vi "Read chat_model.vi"(8 "error in (no error)":errorcluster, 11 "agent_simple_qa in":refnum<class "agent_simple_qa.lvclass">) -> (0 "error out":errorcluster, 2 "abstract_llm_base.lvclass":refnum<class "abstract_llm_base.lvclass">, 3 "agent_simple_qa out":refnum<class "agent_simple_qa.lvclass">)   [LabVIEW 2020, in "agent_simple_qa.lvclass"]
uses:
  agent_simple_qa.lvclass
  models/abstract_llm_base/abstract_llm_base.lvclass
  agent_simple_qa.lvclass/agent_simple_qa.ctl
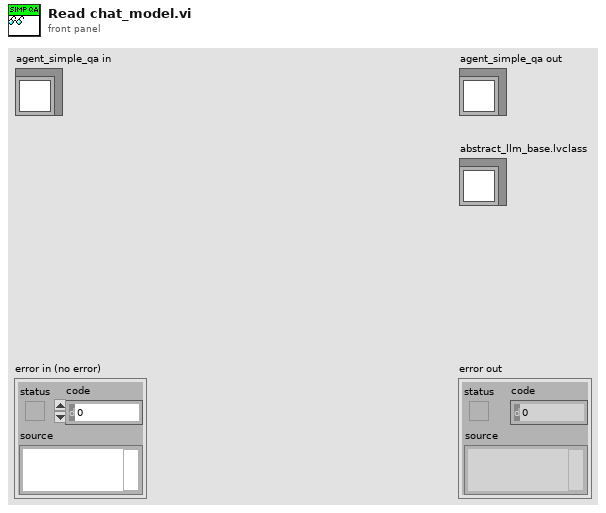
[diagram p1: front panel]
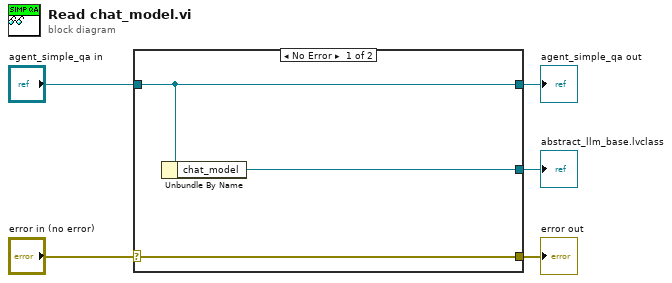
[diagram p0: block diagram]
diagram:
  n1 = case shown="No Error" "error in (no error)" {
    selector: "error in (no error)" -> [w8 w9]
    tunnel: [w8 w9] -> w4
    tunnel: [w7 w10] -> w2
    tunnel: "agent_simple_qa in" -> [w7 w10]
    tunnel: [w6 _] -> w1
    frame No Error {
      n2 = Unbundle By Name(w7) -> ("chat_model"=w6:refnum<class "abstract_llm_base.lvclass">)
    }
    frame Error {
    }
  }
  "error out" <- w4
  "agent_simple_qa out" <- w2
  "abstract_llm_base.lvclass" <- w1
